vi "error if empty buffer.vi"(8 "empty buffer?":bool, 11 "error in (no error)":errorcluster) -> (3 "error out":errorcluster)   [LabVIEW 2021, in "Ring Buffer Strict Accessor.lvlib"]
uses:
  Ring Buffer Strict Accessor.lvlib
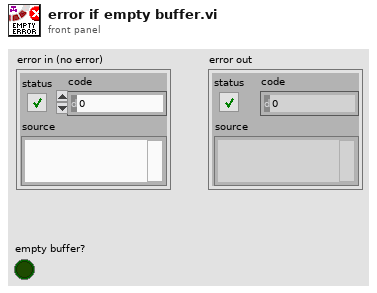
[diagram p1: front panel]
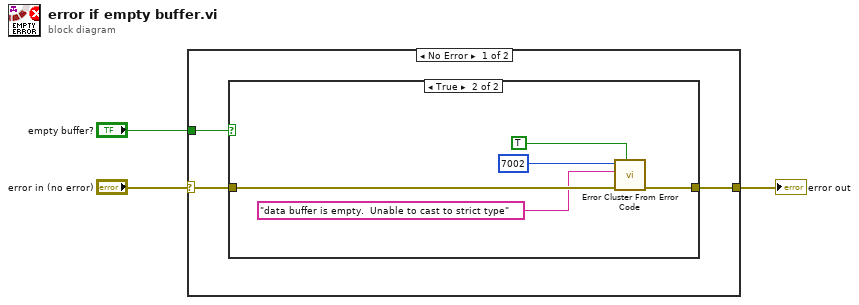
[diagram p0: block diagram]
diagram:
  n1 = case shown="No Error" "error in (no error)" {
    selector: "error in (no error)" -> [w6 w13]
    tunnel: [w5 w13] -> w2
    tunnel: "empty buffer?" -> [w4 _]
    frame No Error {
      n2 = case shown="True" w4 {
        tunnel: w6 -> [w7 w10]
        tunnel: [w7 w9] -> w5
        frame False {
        }
        frame True {
          n3 = call <vilib>:"Error Cluster From Error Code.vi"("show call chain? (False)"=TRUE, "error in (no error)"=w10, "error message (\"\")"="data buffer is empty.  Unable to cast to strict type" ("error message (\"\")"), "error code (0)"=7002) -> ("error out"=w9:errorcluster)  [unwired: 5 in]
        }
      }
    }
    frame Error {
    }
  }
  "error out" <- w2
